vi "load_settings.vi"(8 "error in":errorcluster, 11 "all settings (in)":T1={"Variable Settings"={"Measurements per Iteration"=0, "Local Data Path"=path "", "Experiment description suffix for filename (no spaces please)"="", "Network Data Path"=path "", "Copy data to network"=FALSE, "Measurement Timeout (ms)"=0, "Independent Variables"=[], "Dependent Variables"=[], "Run Test Mode"=FALSE}, "HSDIO Settings"={"Enable HSDIO Pulses"=FALSE, "Resource Name"="PXI1Slot6", "Clock Rate"=20000000.0, "Array of Script Triggers"=[], "Pulse Generation Script"="script script1\n     Generate RedTrap_compress_temp\nend script", "Start Trigger"={"Wait for start trigger?"=FALSE, "source (PFI 0)"="PFI0", "edge (rising)"=12}, "Hardware alignment quantum\n(in samples)"=1, "Inital State"="", "Idle State"="", "Active Channels"="", "Array of Waveforms"=[]}, "DAQmx Pulse Settings"={"Enable DAQmx Pulses"=FALSE, "DAQmx Physical Channels"="", "Clock Rate"=0.0, "units/sec (ms=1000)"=0.0, "Start Trigger"={"Wait for start trigger?"=FALSE, "source"="", "edge"=0}, "Timing Sequence Control"=[]}, "DDS Settings"={"Enable DDS"=FALSE, "Array of DDS Boxes"=[]}, "Camera settings"={"Analog Gain (0-5)"=4, "Exposure Time"=0.01, "EM Gain (0-255)"=0, "Trigger Polarity"="ATP P", "External Trigger Mode"="EMD E", "Scan Speed"="SSP H", "External Trigger Source"="ESC B", "Scan Mode"="SMD N", "Super Pixel Binning\n(if enabled in Scan Mode)"="SPX 1", "Camera Sub-array acquisition region\n(if enabled in scan mode)"={"Left"=0, "Top"=0, "Width"=0, "Height"=0}, "Use camera?"=FALSE, "# image buffers"=100, "shots per measurement"=100, "Force images to U16"=FALSE, "Low Light Sensitivity"="LLS 0", "cooling"="CSW F", "fan"="FAN F", "Frame Grabber acquisition region"={"Left"=0, "Top"=0, "Right"=0, "Bottom"=0}}, "Counter Settings"={"Enable Counters"=FALSE, "Array of Counter Settings"=[]}, "Filter Cluster"={"Counter Filter thresholds"=[], "Data Filters\nROI Minimum Thresholds"=[]}, "Analog Output Parameters"={"Enable Analog Out?"=FALSE, "Physical Channel"="PXI1Slot2/ao0:2", "Minimum Value"=-10.0, "Maximum Value"=10.0, "Samples per second"=0.0, "Total AO Time (seconds)"=0.0, "Start Trigger"={"Wait for start trigger?"=FALSE, "source"="/Dev1/PFI0", "edge"=10280}, "Analog Output Waveforms (channel, time)"=[]}, "Notes"="", "HP83623A Generator Settings Array"=[], "Iteration Graph Settings"={"Plot Regions"="", "Plot Shots"=""}, "PI Piezo Settings"={"Enable"=FALSE, "Array of Piezo Controllers"=[]}, "Andor settings"={"Andor Path"=path "", "Copy any Andor files"=FALSE, "Wait time before copying Andor files (ms)"=0}, "Measurement Chart Settings"={"Which regions to plot (comma separated)"="", "Which shot to plot"=0}, "HP8662A Synthesized Signal Generator Array"=[], "HP83712B Synthesized CW Generator Array"=[], "TTL input"={"Enable"=FALSE, "lines"=""}} {"Variable Settings"."Independent Variables"."# steps" min=1 step=1; "Variable Settings"."Measurements per Iteration" min=1 step=1; "HSDIO Settings"."Hardware alignment quantum\n(in samples)" min=1 step=1; "HSDIO Settings"."Array of Script Triggers"."level" items=["High Level"=34, "Low Level"=35]; "HSDIO Settings"."Array of Script Triggers"."edge" items=["Rising Edge"=12, "Falling Edge"=13]; "HSDIO Settings"."Start Trigger"."edge (rising)" items=["Rising Edge"=12, "Falling Edge"=13]; "HSDIO Settings"."Clock Rate" min=0.0 max=200000000.0 format="%.2p"; "DAQmx Pulse Settings"."Start Trigger"."edge" items=["Rising"=10280, "Falling"=10171]; "DAQmx Pulse Settings"."Clock Rate" min=0.0 max=200000000.0 format="%.2p"; "Camera settings"."Frame Grabber acquisition region"."Bottom" max=512 step=1; "Camera settings"."Frame Grabber acquisition region"."Right" max=512 step=1; "Camera settings"."Frame Grabber acquisition region"."Top" max=512 step=1; "Camera settings"."Frame Grabber acquisition region"."Left" max=512 step=1; "Camera settings"."shots per measurement" min=0 step=1; "Camera settings"."# image buffers" min=0 step=1; "Camera settings"."Camera Sub-array acquisition region\n(if enabled in scan mode)"."Height" min=16 max=512 step=16; "Camera settings"."Camera Sub-array acquisition region\n(if enabled in scan mode)"."Width" min=16 max=512 step=16; "Camera settings"."Camera Sub-array acquisition region\n(if enabled in scan mode)"."Top" max=496 step=16; "Camera settings"."Camera Sub-array acquisition region\n(if enabled in scan mode)"."Left" max=496 step=16; "Camera settings"."Analog Gain (0-5)" max=5 step=1; "Counter Settings"."Array of Counter Settings"."Binwidth (ms)" format="%0.2f"; "Analog Output Parameters"."Start Trigger"."edge" items=["Rising"=10280, "Falling"=10171]; "Analog Output Parameters"."Maximum Value" format="%0.2f"; "Analog Output Parameters"."Minimum Value" format="%0.2f"}) -> (0 "error out":errorcluster, 3 "all settings":T1={"Variable Settings"={"Measurements per Iteration"=0, "Local Data Path"=path "", "Experiment description suffix for filename (no spaces please)"="", "Network Data Path"=path "", "Copy data to network"=FALSE, "Measurement Timeout (ms)"=0, "Independent Variables"=[], "Dependent Variables"=[], "Run Test Mode"=FALSE}, "HSDIO Settings"={"Enable HSDIO Pulses"=FALSE, "Resource Name"="PXI1Slot6", "Clock Rate"=20000000.0, "Array of Script Triggers"=[], "Pulse Generation Script"="script script1\n     Generate RedTrap_compress_temp\nend script", "Start Trigger"={"Wait for start trigger?"=FALSE, "source (PFI 0)"="PFI0", "edge (rising)"=12}, "Hardware alignment quantum\n(in samples)"=1, "Inital State"="", "Idle State"="", "Active Channels"="", "Array of Waveforms"=[]}, "DAQmx Pulse Settings"={"Enable DAQmx Pulses"=FALSE, "DAQmx Physical Channels"="", "Clock Rate"=0.0, "units/sec (ms=1000)"=0.0, "Start Trigger"={"Wait for start trigger?"=FALSE, "source"="", "edge"=0}, "Timing Sequence Control"=[]}, "DDS Settings"={"Enable DDS"=FALSE, "Array of DDS Boxes"=[]}, "Camera settings"={"Analog Gain (0-5)"=4, "Exposure Time"=0.01, "EM Gain (0-255)"=0, "Trigger Polarity"="ATP P", "External Trigger Mode"="EMD E", "Scan Speed"="SSP H", "External Trigger Source"="ESC B", "Scan Mode"="SMD N", "Super Pixel Binning\n(if enabled in Scan Mode)"="SPX 1", "Camera Sub-array acquisition region\n(if enabled in scan mode)"={"Left"=0, "Top"=0, "Width"=0, "Height"=0}, "Use camera?"=FALSE, "# image buffers"=100, "shots per measurement"=100, "Force images to U16"=FALSE, "Low Light Sensitivity"="LLS 0", "cooling"="CSW F", "fan"="FAN F", "Frame Grabber acquisition region"={"Left"=0, "Top"=0, "Right"=0, "Bottom"=0}}, "Counter Settings"={"Enable Counters"=FALSE, "Array of Counter Settings"=[]}, "Filter Cluster"={"Counter Filter thresholds"=[], "Data Filters\nROI Minimum Thresholds"=[]}, "Analog Output Parameters"={"Enable Analog Out?"=FALSE, "Physical Channel"="PXI1Slot2/ao0:2", "Minimum Value"=-10.0, "Maximum Value"=10.0, "Samples per second"=0.0, "Total AO Time (seconds)"=0.0, "Start Trigger"={"Wait for start trigger?"=FALSE, "source"="/Dev1/PFI0", "edge"=10280}, "Analog Output Waveforms (channel, time)"=[]}, "Notes"="", "HP83623A Generator Settings Array"=[], "Iteration Graph Settings"={"Plot Regions"="", "Plot Shots"=""}, "PI Piezo Settings"={"Enable"=FALSE, "Array of Piezo Controllers"=[]}, "Andor settings"={"Andor Path"=path "", "Copy any Andor files"=FALSE, "Wait time before copying Andor files (ms)"=0}, "Measurement Chart Settings"={"Which regions to plot (comma separated)"="", "Which shot to plot"=0}, "HP8662A Synthesized Signal Generator Array"=[], "HP83712B Synthesized CW Generator Array"=[], "TTL input"={"Enable"=FALSE, "lines"=""}} {"Variable Settings"."Independent Variables"."# steps" min=1 step=1; "Variable Settings"."Measurements per Iteration" min=1 step=1; "HSDIO Settings"."Hardware alignment quantum\n(in samples)" min=1 step=1; "HSDIO Settings"."Array of Script Triggers"."level" items=["High Level"=34, "Low Level"=35]; "HSDIO Settings"."Array of Script Triggers"."edge" items=["Rising Edge"=12, "Falling Edge"=13]; "HSDIO Settings"."Start Trigger"."edge (rising)" items=["Rising Edge"=12, "Falling Edge"=13]; "HSDIO Settings"."Clock Rate" min=0.0 max=200000000.0 format="%.2p"; "DAQmx Pulse Settings"."Start Trigger"."edge" items=["Rising"=10280, "Falling"=10171]; "DAQmx Pulse Settings"."Clock Rate" min=0.0 max=200000000.0 format="%.2p"; "Camera settings"."Frame Grabber acquisition region"."Bottom" max=512 step=1; "Camera settings"."Frame Grabber acquisition region"."Right" max=512 step=1; "Camera settings"."Frame Grabber acquisition region"."Top" max=512 step=1; "Camera settings"."Frame Grabber acquisition region"."Left" max=512 step=1; "Camera settings"."shots per measurement" min=0 step=1; "Camera settings"."# image buffers" min=0 step=1; "Camera settings"."Camera Sub-array acquisition region\n(if enabled in scan mode)"."Height" min=16 max=512 step=16; "Camera settings"."Camera Sub-array acquisition region\n(if enabled in scan mode)"."Width" min=16 max=512 step=16; "Camera settings"."Camera Sub-array acquisition region\n(if enabled in scan mode)"."Top" max=496 step=16; "Camera settings"."Camera Sub-array acquisition region\n(if enabled in scan mode)"."Left" max=496 step=16; "Camera settings"."Analog Gain (0-5)" max=5 step=1; "Counter Settings"."Array of Counter Settings"."Binwidth (ms)" format="%0.2f"; "Analog Output Parameters"."Start Trigger"."edge" items=["Rising"=10280, "Falling"=10171]; "Analog Output Parameters"."Maximum Value" format="%0.2f"; "Analog Output Parameters"."Minimum Value" format="%0.2f"})   [LabVIEW 2013, in "Experiment.lvclass"]
doc: "This .vi allows loading settings from .xml files.\n\nThe current settings must be passed in, so that they can be preserved if some sections are not overwritten.\n\nThe user selects a .xml file using the dialog.\n\nFirst the selected file is checked to see which types of settings it contains. The user is then allowed to pick from those in \"Load What?\".\n\nThe selected sections are then extracted as xml nodes, which are passed to individual .vi's to parse. The created cluster is then written back to the front panel settings via the outputs from this .vi\n\nMTL 2012 Dec 30"
uses:
  Experiment/Experiment.lvclass
  <vilib>/xml/NI_XML.lvlib
  <vilib>/xml/Load XML File.vi
  <vilib>/xml/Close Reference(Node).vi
  ExperimentVariables/ExperimentVariables.lvclass
  HSDIO/HSDIO.lvclass
  DAQmx_pulse_out/DAQmx_pulse_out.lvclass
  DDS/DDS.lvclass
  Camera/Hamamatsu_C9100-13/Hamamatsu_C9100-13.lvclass
  Counter/Counter.lvclass
  Analog_output/Analog_Output.lvclass
  GPIB/GPIB.lvclass
  PI_piezo/PI_Piezo.lvclass
  Camera/Hamamatsu_C9100-13/camera_setup.ctl
  ExperimentVariables/Variable_Settings.ctl
  Analog_output/AO_settings.ctl
  filters/filters.ctl
  Counter/Counter_Settings_Control.ctl
  <vilib>/ni845x/ni845x.llb/ni845xControl.ctl
  DDS drivers v3/DDS_box_device_reference.ctl
  DDS drivers v3/DDS RAM mode.ctl
  DDS drivers v3/DDS_box_cluster.ctl
  DDS drivers v3/Array_of_DDS_Boxes.ctl
  DDS/DDS_Settings_Cluster.ctl
  DAQmx_pulse_out/settings.ctl
  <instrlib>/niHSDIO/niHSDIO.llb/niHSDIO_ctl Trigger Source Values (Ring).ctl
  <instrlib>/niHSDIO/niHSDIO.llb/niHSDIO_ctl Trigger DigEdge - Edge Values (Ring).ctl
  <instrlib>/niHSDIO/niHSDIO.llb/niHSDIO_ctl Trigger Script - trigID Values (Ring).ctl
  <instrlib>/niHSDIO/niHSDIO.llb/niHSDIO_ctl Trigger DigLvl - Level Values (Ring).ctl
  HSDIO/HSDIO_settings.ctl
  all_settings.ctl
  GPIB/HP83623A_RF_Generator/HP83623A_array.ctl
  GPIB/HP83623A_RF_Generator/HP83623A_RF_Generator.lvclass
  PI_piezo/settings.ctl
  Camera/Andor/Andor_settings.ctl
  gui/measurement_graph.ctl
  GPIB/RF_Generator_settings.ctl
  GPIB/RF_Generator_settings_array.ctl
  DDS drivers v3/DDS_profile.ctl
  DDS drivers v3/DDS_channel.ctl
  DDS drivers v3/array_of_DDS_profiles.ctl
  DDS drivers v3/array_of_DDS_channels.ctl
  TTL_input/TTL_input_settings.ctl
  TTL_input/TTL_input.lvclass
  HSDIO/waveform.ctl
  PI_piezo/piezo_channel.ctl
  PI_piezo/piezo_controller.ctl
  GPIB/HP83623A_RF_Generator/HP83623A.ctl
panel:
  # "Parameters will be evaluated once at the beginning of the experiment from top to bottom, \nso any parameter may depend on all those above it.\nVariables will be evaluated each iteration.\nParameters and Variables may be used in various other experiment settings, as noted.\nSee LabView Help -> Formula Node and Expression Node Functions for a list of available functions."
  # "Regions of Interest -->"
  # "Shots\n   |\n  V"
  # "Counters -->"
  # "Counter\n    bins\n       |\n      V"
  # "Parameters will be evaluated once at the beginning of the experiment from top to bottom, \nso any parameter may depend on all those above it.\nVariables will be evaluated each iteration.\nParameters and Variables may be used in various other experiment settings, as noted.\nSee LabView Help -> Formula Node and Expression Node Functions for a list of available functions."
  # "Regions of Interest -->"
  # "Shots\n   |\n  V"
  # "Counters -->"
  # "Counter\n    bins\n       |\n      V"
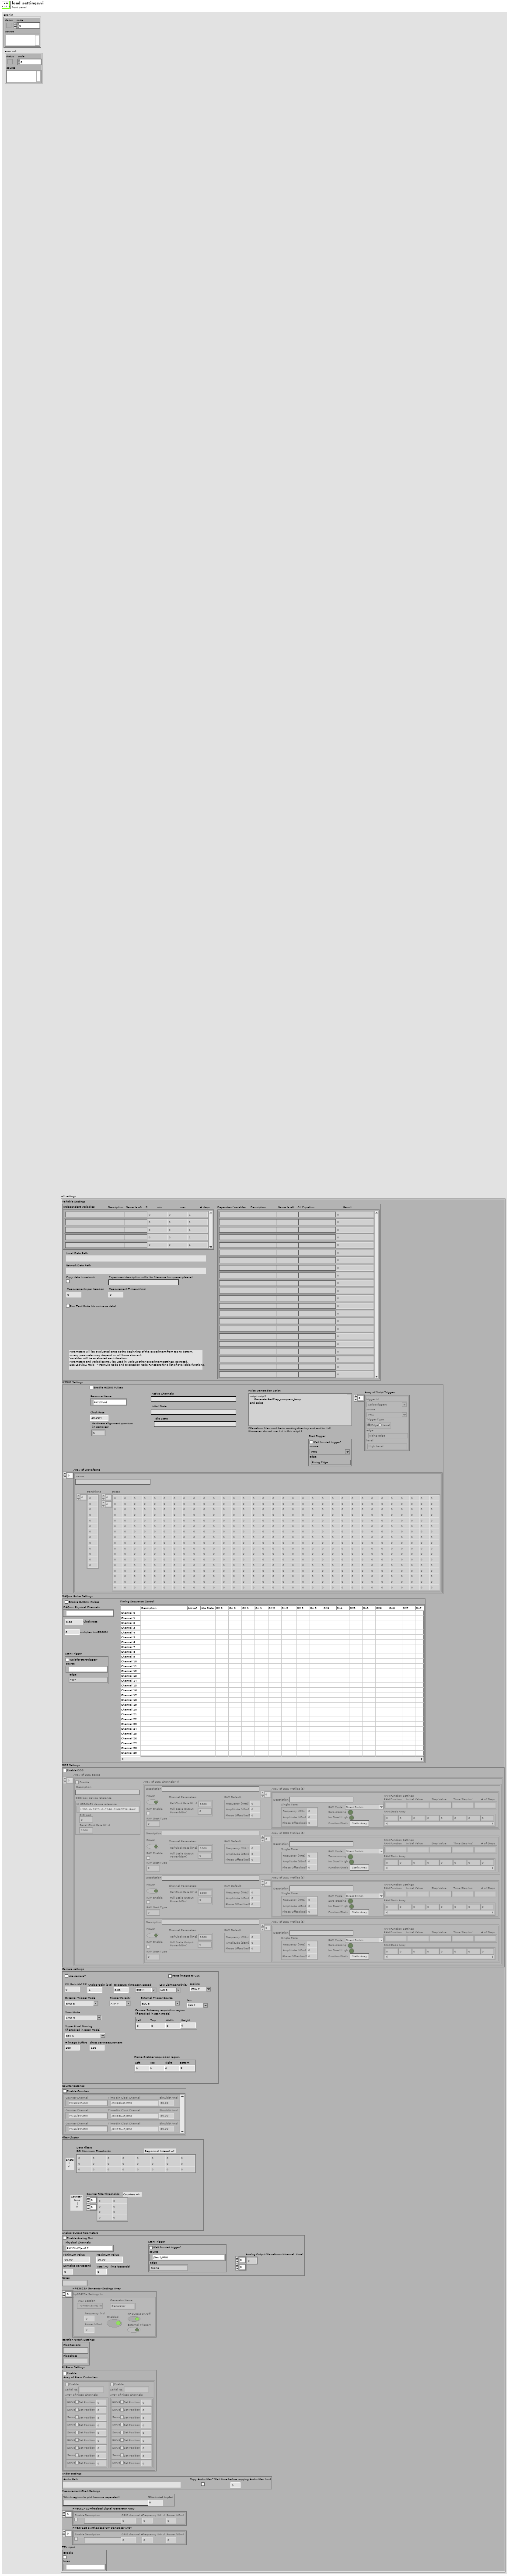
[diagram p1: front panel]
types:
  T1 = typedef "all_settings.ctl" = cluster{"Variable Settings":T2, "HSDIO Settings":T3, "DAQmx Pulse Settings":T9, "DDS Settings":T10, "Camera settings":T20, "Counter Settings":T21, "Filter Cluster":T22, "Analog Output Parameters":T23, "Notes":string, "HP83623A Generator Settings Array":T24, "Iteration Graph Settings":cluster{"Plot Regions":string, "Plot Shots":string}, "PI Piezo Settings":T26, "Andor settings":T29, "Measurement Chart Settings":T30, "HP8662A Synthesized Signal Generator Array":T31, "HP83712B Synthesized CW Generator Array":T31, "TTL input":T33}
  T2 = typedef "ExperimentVariables.lvclass/Variable_Settings.ctl" = cluster{"Measurements per Iteration":i32, "Local Data Path":path, "Experiment description suffix for filename (no spaces please)":string, "Network Data Path":path, "Copy data to network":bool, "Measurement Timeout (ms)":u32, "Independent Variables":cluster{"Description":string, "Name (a,a0...a9)":string, "min":dbl, "max":dbl, "# steps":u32}[], "Dependent Variables":cluster{"Description":string, "Name (a,a0...a9)":string, "Equation":string, "Result":dbl}[], "Run Test Mode":bool}
  T3 = typedef "HSDIO.lvclass/HSDIO_settings.ctl" = cluster{"Enable HSDIO Pulses":bool, "Resource Name":refnum<k15>, "Clock Rate":dbl, "Array of Script Triggers":cluster{"trigger id (script trigger 0)":T4, "source (PFI 0)":T5, "Trigger Type":enum32{"Edge", "Level"}, "edge":T6, "level":T7}[], "Pulse Generation Script":string, "Start Trigger":cluster{"Wait for start trigger?":bool, "source (PFI 0)":T5, "edge (rising)":T6}, "Hardware alignment quantum\n(in samples)":u16, "Inital State":string, "Idle State":string, "Active Channels":string, "Array of Waveforms":T8[]}
  T4 = typedef "niHSDIO_ctl Trigger Script - trigID Values (Ring).ctl" = string
  T5 = typedef "niHSDIO_ctl Trigger Source Values (Ring).ctl" = string
  T6 = typedef "niHSDIO_ctl Trigger DigEdge - Edge Values (Ring).ctl" = i32
  T7 = typedef "niHSDIO_ctl Trigger DigLvl - Level Values (Ring).ctl" = i32
  T8 = typedef "HSDIO.lvclass/waveform.ctl" = cluster{"name":string, "transitions":u32[], "states":u8[][]}
  T9 = typedef "DAQmx_pulse_out.lvclass/settings.ctl" = cluster{"Enable DAQmx Pulses":bool, "DAQmx Physical Channels":tag, "Clock Rate":dbl, "units/sec (ms=1000)":dbl, "Start Trigger":cluster{"Wait for start trigger?":bool, "source":tag, "edge":i32}, "Timing Sequence Control":string[][]}
  T10 = typedef "DDS_Settings_Cluster.ctl" = cluster{"Enable DDS":bool, "Array of DDS Boxes":T11}
  T11 = typedef "Array_of_DDS_Boxes.ctl" = T12[]
  T12 = typedef "DDS_box_cluster.ctl" = cluster{"DDS box device reference":T13, "Array of DDS Channels (4)":T15, "Enable":bool, "Description":string}
  T13 = typedef "DDS_box_device_reference.ctl" = cluster{"NI USB-8451 device reference":T14, "DIO port":u8, "Serial Clock Rate [kHz]":u16}
  T14 = typedef "ni845xControl.ctl" = refnum<k21>
  T15 = typedef "DDS.lvclass/array_of_DDS_channels.ctl" = T16[]
  T16 = typedef "DDS.lvclass/DDS_channel.ctl" = cluster{"Power":bool, "Channel Parameters":cluster{"Ref Clock Rate [kHz]":dbl, "Full Scale Output\nPower [dBm]":dbl}, "RAM Enable":bool, "RAM Dest Type":u8, "RAM Default":cluster{"Frequency [MHz]":dbl, "Amplitude [dBm]":dbl, "Phase Offset [rad]":dbl}, "Array of DDS Profiles (8)":T17, "Description":string}
  T17 = typedef "DDS.lvclass/array_of_DDS_profiles.ctl" = T18[]
  T18 = typedef "DDS_profile.ctl" = cluster{"Single Tone":cluster{"Frequency [MHz]":dbl, "Amplitude [dBm]":dbl, "Phase Offset [rad]":dbl}, "RAM Mode ":T19, "Zero-crossing":bool, "No Dwell High":bool, "Function/Static":bool, "RAM Function Settings":string[], "RAM Static Array":dbl[], "Description":string}
  T19 = typedef "DDS RAM mode.ctl" = enum16{"Direct Switch", "Ramp Up", "Bidirectional Ramp", "Continuous Bidirectional Ramp", "Continuous Recirculate", "Direct Switch 2", "Direct Switch 3", "Direct Switch 4"}
  T20 = typedef "Hamamatsu_C9100-13.lvclass/camera_setup.ctl" = cluster{"Analog Gain (0-5)":u8, "Exposure Time":dbl, "EM Gain (0-255)":u8, "Trigger Polarity":string, "External Trigger Mode":string, "Scan Speed":string, "External Trigger Source":string, "Scan Mode":string, "Super Pixel Binning\n(if enabled in Scan Mode)":string, "Camera Sub-array acquisition region\n(if enabled in scan mode)":cluster{"Left":u16, "Top":u16, "Width":u16, "Height":u16}, "Use camera?":bool, "# image buffers":i32, "shots per measurement":i32, "Force images to U16":bool, "Low Light Sensitivity":string, "cooling":string, "fan":string, "Frame Grabber acquisition region":cluster{"Left":i32, "Top":i32, "Right":i32, "Bottom":i32}}
  T21 = typedef "Counter.lvclass/Counter_Settings_Control.ctl" = cluster{"Enable Counters":bool, "Array of Counter Settings":cluster{"Counter Channel":tag, "Time-Bin Clock Channel":tag, "Binwidth (ms)":dbl}[]}
  T22 = typedef "filters.ctl" = cluster{"Counter Filter thresholds":u32[][], "Data Filters\nROI Minimum Thresholds":u64[][]}
  T23 = typedef "Analog_Output.lvclass/AO_settings.ctl" = cluster{"Enable Analog Out?":bool, "Physical Channel":tag, "Minimum Value":dbl, "Maximum Value":dbl, "Samples per second":dbl, "Total AO Time (seconds)":dbl, "Start Trigger":cluster{"Wait for start trigger?":bool, "source":tag, "edge":i32}, "Analog Output Waveforms (channel, time)":dbl[][]}
  T24 = typedef "HP83623A_RF_Generator.lvclass/HP83623A_array.ctl" = T25[]
  T25 = typedef "HP83623A_RF_Generator.lvclass/HP83623A.ctl" = cluster{"Frequency (Hz)":dbl, "Power (dBm)":dbl, "Enabled":bool, "initialized":bool, "RF Output On/Off":bool, "External Trigger?":bool, "VISA Session":refnum<visa-resource-name>, "Generator Name":string}
  T26 = typedef "PI_Piezo.lvclass/settings.ctl" = cluster{"Enable":bool, "Array of Piezo Controllers":T27[]}
  T27 = typedef "PI_Piezo.lvclass/piezo_controller.ctl" = cluster{"Enable":bool, "Serial No.":string, "Array of Piezo Channels":T28[]}
  T28 = typedef "PI_Piezo.lvclass/piezo_channel.ctl" = cluster{"Servo":bool, "Set Position":dbl}
  T29 = typedef "Andor_settings.ctl" = cluster{"Andor Path":path, "Copy any Andor files":bool, "Wait time before copying Andor files (ms)":u16}
  T30 = typedef "measurement_graph.ctl" = cluster{"Which regions to plot (comma separated)":string, "Which shot to plot":u8}
  T31 = typedef "GPIB.lvclass/RF_Generator_settings_array.ctl" = T32[]
  T32 = typedef "GPIB.lvclass/RF_Generator_settings.ctl" = cluster{"Enable":bool, "Description":string, "GPIB channel #":u8, "Frequency (MHz)":dbl, "Power (dBm)":dbl}
  T33 = typedef "TTL_input.lvclass/TTL_input_settings.ctl" = cluster{"Enable":bool, "lines":tag}
  T34 = cluster{"Set none to load by default.":bool, "XPath expression":string}
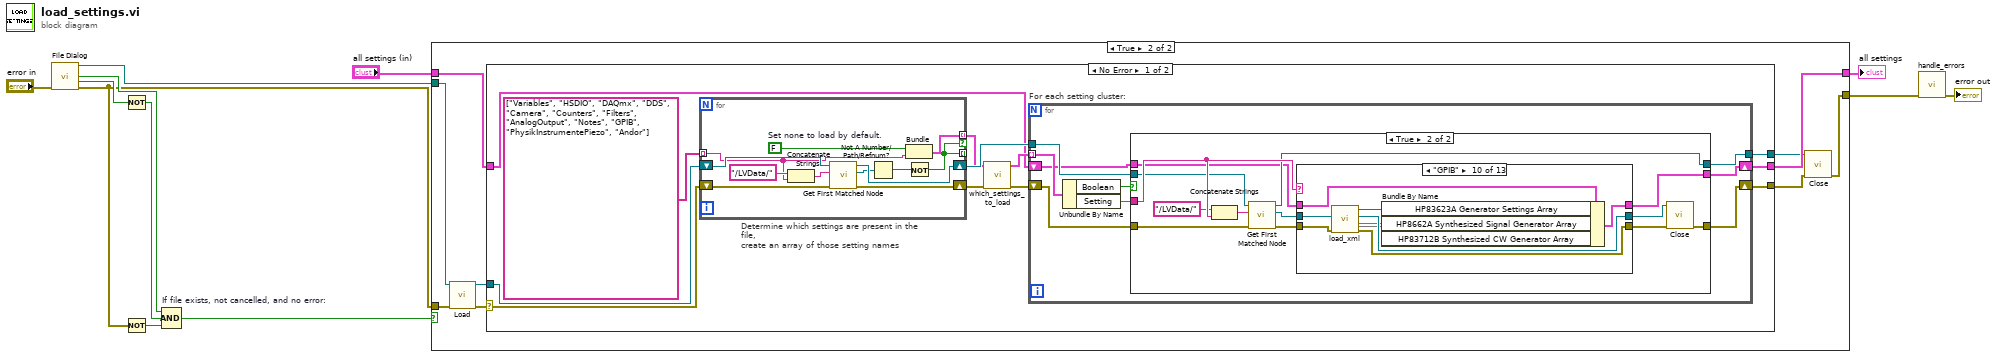
[diagram p0: block diagram]
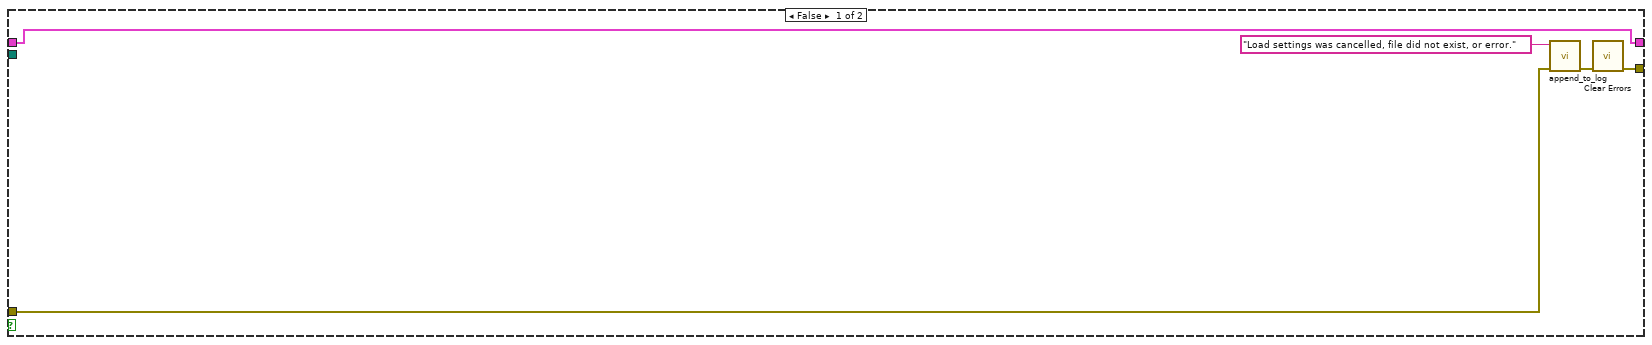
[diagram p2: hidden frame]
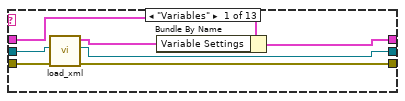
[diagram p4: hidden frame]
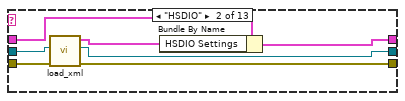
[diagram p5: hidden frame]
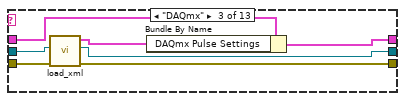
[diagram p6: hidden frame]
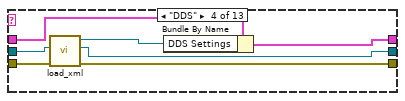
[diagram p7: hidden frame]
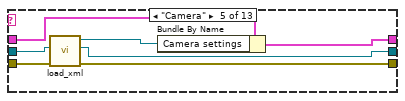
[diagram p8: hidden frame]
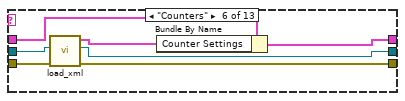
[diagram p9: hidden frame]
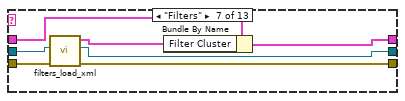
[diagram p10: hidden frame]
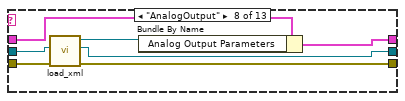
[diagram p11: hidden frame]
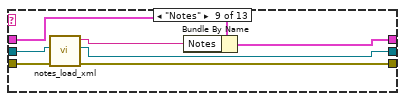
[diagram p12: hidden frame]
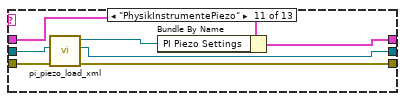
[diagram p13: hidden frame]
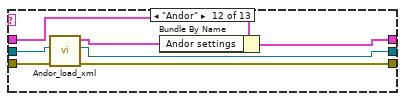
[diagram p14: hidden frame]
diagram:
  n1 = call "File Dialog"("error in"="error in") -> ("selected path"=w12:path, "exists"=w6:bool, "cancelled"=w5:bool, "error out"=w2:errorcluster)  [unwired: 11 in]
  n2 = Not(x=w5) -> (.not. x?=w4:bool)
  n3 = Not(x=w2) -> (.not. x?=w1:bool)
  n4 = Compound Arithmetic op=AND "If file exists, not cancelled, and no error:"(w6, w4, w1) -> (w3:bool)
  n5 = case shown="True" w3 {
    tunnel: w12 -> [_ w26]
    tunnel: [w16 w19] -> w7
    tunnel: "all settings (in)" -> [w17 w23]
    tunnel: [w17 w22] -> w8
    tunnel: w2 -> [w14 w18]
    frame False {
      n6 = call "append_to_log.vi"("error in"=w14, "string"="Load settings was cancelled, file did not exist, or error.") -> ("error out"=w13:errorcluster)  [unwired: 9 in]
      n7 = call <vilib>:"Clear Errors.vi"("error in (no error)"=w13) -> ("error out"=w16:errorcluster)  [unwired: 6 in]
    }
    frame True {
      n8 = call-poly <vilib>:"Load.vi"("path to XML document"=w26, "error in (no error)"=w18) -> ("DOM document out"=w25:refnum<k20>, "error out"=w24:errorcluster)  [unwired: 11 in, 1 out]
      n9 = case shown="No Error" w24 {
        selector: w24 -> [w30 w167]
        tunnel: w25 -> [w36 w165]
        tunnel: [w31 w167] -> w20
        tunnel: [w29 w165] -> w21
        tunnel: w23 -> [w28 w166]
        tunnel: [w27 w166] -> w22
        frame No Error {
          n10 = for "Determine which settings are present in the file,\ncreate an array of those setting names" {
            tunnel: string[] ["Variables", "HSDIO", "DAQmx", "DDS", "Camera", "Counters", "Filters", "AnalogOutput", "Notes", "GPIB", "PhysikInstrumentePiezo", "Andor"] -> [w156] mode=indexing
            shift-right: [w162] -> w34
            shift-left: w36 -> [w161]
            shift-right: [w157] -> w37
            shift-left: w30 -> [w158]
            tunnel: [w155] -> w32 mode=indexing if=w153
            tunnel: [w153] -> _ mode=indexing
            w154 = FALSE  # Set none to load by default.
            n11 = Concatenate Strings("/LVData/" ("XPath expression"), w156) -> (w163:string)
            n12 = call <vilib>:"Get First Matched Node.vi"("error in (no error)"=w158, "XPath expression"=w163, "node in"=w161) -> ("error out"=w157:errorcluster, "node result"=w160:refnum<k20>, "node out"=w162:refnum<k20>)  [unwired: 6 in]
            n13 = Not A Number/Path/Refnum?(number/path/refnum=w160) -> (NaN/Path/Refnum?=w159:bool)
            n14 = Bundle("Set none to load by default."=w154, "XPath expression"=w156) -> (w155:T34)  [unwired: 1 in]
            n15 = Not(x=w159) -> (.not. x?=w153:bool)
          }
          n16 = call "which_settings_to_load.vi"("error in (no error)"=w37, "Which settings to load (in)"=w32) -> ("error out"=w33:errorcluster, "Which settings to load"=w35:cluster{"Boolean":bool, "Setting":string}[])  [unwired: 8 in]
          n17 = for "For each setting cluster:" {
            tunnel: w35 -> [w47] mode=indexing
            tunnel: w34 -> [w44]
            shift-right: [w43] -> w31
            shift-left: w33 -> [w42]
            tunnel: [w41] -> w29
            shift-right: [w39] -> w27
            shift-left: w28 -> [w40]
            n18 = Unbundle By Name(w47) -> ("Boolean"=w46:bool, "Setting"=w45:string)
            n19 = case shown="True" w46 {
              tunnel: w45 -> [_ w63]
              tunnel: w44 -> [w49 w60]
              tunnel: [w50 w55] -> w43
              tunnel: w42 -> [w50 w59]
              tunnel: [w49 w58] -> w41
              tunnel: w40 -> [w48 w54]
              tunnel: [w48 w53] -> w39
              frame False {
              }
              frame True {
                n20 = Concatenate Strings("/LVData/" ("XPath expression"), w63) -> (w61:string)
                n21 = call <vilib>:"Get First Matched Node.vi"("error in (no error)"=w59, "XPath expression"=w61, "node in"=w60) -> ("error out"=w51:errorcluster, "node result"=w52:refnum<k20>, "node out"=w58:refnum<k20>)  [unwired: 6 in]
                n22 = case shown="\"GPIB\"" w63 {
                  tunnel: w51 -> [w70 w73 w82 w87 w94 w101 w109 w117 w122 w131 w139 w147 w152]
                  tunnel: [w64 w71 w81 w86 w93 w99 w108 w116 w121 w130 w138 w146 w152] -> w56
                  tunnel: w52 -> [w69 w75 w79 w89 w96 w103 w110 w115 w124 w133 w140 w143 w151]
                  tunnel: [w68 w74 w78 w88 w95 w102 w106 w114 w123 w132 w137 w145 w151] -> w57
                  tunnel: w54 -> [w67 w76 w84 w91 w98 w105 w112 w119 w126 w135 w142 w149 w150]
                  tunnel: [w65 w77 w83 w90 w97 w104 w111 w118 w125 w134 w141 w148 w150] -> w53
                  frame "Variables" {
                    n23 = call "load_xml.vi"("error in"=w70, "child node in"=w69) -> ("error out"=w64:errorcluster, "child node out"=w68:refnum<k20>, "Variable Settings"=w66:T2)  [unwired: 7 in]
                    n24 = Bundle By Name(cluster=w67, "Variable Settings"=w66) -> (w65:T1)
                  }
                  frame "HSDIO" {
                    n25 = call "load_xml.vi"("error in"=w73, "child node in"=w75) -> ("error out"=w71:errorcluster, "child node out"=w74:refnum<k20>, "HSDIO Settings"=w72:T3)  [unwired: 7 in]
                    n26 = Bundle By Name(cluster=w76, "HSDIO Settings"=w72) -> (w77:T1)
                  }
                  frame "DAQmx" {
                    n27 = call "load_xml.vi"("error in"=w82, "child node in"=w79) -> ("error out"=w81:errorcluster, "child node out"=w78:refnum<k20>, "DAQmx Pulse Settings"=w80:T9)  [unwired: 7 in]
                    n28 = Bundle By Name(cluster=w84, "DAQmx Pulse Settings"=w80) -> (w83:T1)
                  }
                  frame "DDS" {
                    n29 = call "load_xml.vi"("error in"=w87, "child node in"=w89) -> ("error out"=w86:errorcluster, "child node out"=w88:refnum<k20>, "DDS.lvclass"=w85:refnum<class "DDS.lvclass">)  [unwired: 7 in]
                    n30 = Bundle By Name(cluster=w91, "DDS Settings"=w85) -> (w90:T1)
                  }
                  frame "Camera" {
                    n31 = call "load_xml.vi"("error in"=w94, "child node in"=w96) -> ("error out"=w93:errorcluster, "child node out"=w95:refnum<k20>, "Hamamatsu_C9100-13.lvclass"=w92:refnum<class "Hamamatsu_C9100-13.lvclass">)  [unwired: 7 in]
                    n32 = Bundle By Name(cluster=w98, "Camera settings"=w92) -> (w97:T1)
                  }
                  frame "Counters" {
                    n33 = call "load_xml.vi"("error in"=w101, "child node in"=w103) -> ("error out"=w99:errorcluster, "child node out"=w102:refnum<k20>, "Counter Settings"=w100:T21)  [unwired: 7 in]
                    n34 = Bundle By Name(cluster=w105, "Counter Settings"=w100) -> (w104:T1)
                  }
                  frame "Filters" {
                    n35 = call "filters_load_xml.vi"("error in"=w109, "child node in"=w110) -> ("error out"=w108:errorcluster, "child node out"=w106:refnum<k20>, "Filter Settings"=w107:T22)  [unwired: 7 in]
                    n36 = Bundle By Name(cluster=w112, "Filter Cluster"=w107) -> (w111:T1)
                  }
                  frame "AnalogOutput" {
                    n37 = call "load_xml.vi"("error in"=w117, "child node in"=w115) -> ("error out"=w116:errorcluster, "child node out"=w114:refnum<k20>, "Analog_Output.lvclass"=w113:refnum<class "Analog_Output.lvclass">)  [unwired: 7 in]
                    n38 = Bundle By Name(cluster=w119, "Analog Output Parameters"=w113) -> (w118:T1)
                  }
                  frame "Notes" {
                    n39 = call "notes_load_xml.vi"("error in"=w122, "child node in"=w124) -> ("error out"=w121:errorcluster, "child node out"=w123:refnum<k20>, "notes"=w120:string)  [unwired: 7 in]
                    n40 = Bundle By Name(cluster=w126, "Notes"=w120) -> (w125:T1)
                  }
                  frame "GPIB" {
                    n41 = call "load_xml.vi"("error in"=w131, "child node in"=w133) -> ("error out"=w130:errorcluster, 1:w128, "child node out"=w132:refnum<k20>, "GPIB"=w129:refnum<class "GPIB.lvclass">, 4:w127)  [unwired: 5 in]
                    n42 = Bundle By Name(cluster=w135, "HP83623A Generator Settings Array"=w129, "HP8662A Synthesized Signal Generator Array"=w128, "HP83712B Synthesized CW Generator Array"=w127) -> (w134:T1)
                  }
                  frame "PhysikInstrumentePiezo" {
                    n43 = call "pi_piezo_load_xml.vi"("error in"=w139, "child node in"=w140) -> ("error out"=w138:errorcluster, "child node out"=w137:refnum<k20>, "PI_Piezo"=w136:refnum<class "PI_Piezo.lvclass">)  [unwired: 7 in]
                    n44 = Bundle By Name(cluster=w142, "PI Piezo Settings"=w136) -> (w141:T1)
                  }
                  frame "Andor" {
                    n45 = call "Andor_load_xml.vi"("error in"=w147, "child node in"=w143) -> ("error out"=w146:errorcluster, "child node out"=w145:refnum<k20>, "Andor settings"=w144:T29)  [unwired: 7 in]
                    n46 = Bundle By Name(cluster=w149, "Andor settings"=w144) -> (w148:T1)
                  }
                  frame "None", Default {
                  }
                }
                n47 = call-poly <vilib>:"Close.vi"("error in (no error)"=w56, "node"=w57) -> ("error out"=w55:errorcluster)  [unwired: 7 in]
              }
            }
          }
        }
        frame Error {
        }
      }
      n48 = call-poly <vilib>:"Close.vi"("error in (no error)"=w20, "node"=w21) -> ("error out"=w19:errorcluster)  [unwired: 7 in]
    }
  }
  "all settings" <- w8
  n49 = call "handle_errors.vi"("error in (no error)"=w7) -> ("error out"=→"error out":errorcluster)  [unwired: 10 in]
